vi "Send Message Log Ready String to Debug Client.vi"(8 "error in (no error)":errorcluster, 10 "DC_UID":T1, 11 "DS TCP Server in":refnum<class "DS TCP Server.lvclass">) -> (0 "error out":errorcluster, 3 "DS TCP Server out":refnum<class "DS TCP Server.lvclass">)   [LabVIEW 2017, in "DS TCP Server.lvlib" / "DS TCP Server.lvclass"]
uses:
  DS TCP Server.lvclass
  Common VIs/DC_UID.ctl
  C:/Program Files (x86)/National Instruments/LabVIEW 2017/vi.lib/addons/_Workers/Library/Classes/Worker/Worker.lvclass
  rqp_Send Data to Debug Client.ctl
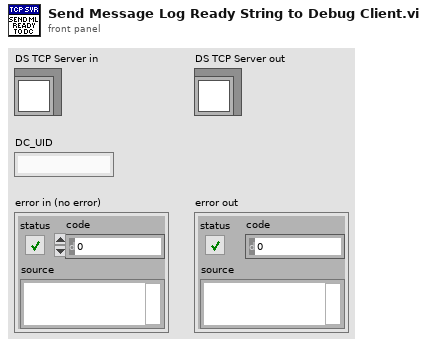
[diagram p1: front panel]
types:
  T1 = typedef "DC_UID.ctl" = string
  T2 = typedef "DS TCP Server.lvlib/DS TCP Server.lvclass/rqp_Send Data to Debug Client.ctl" = cluster{"DC_UID":T1, "String to send":string}
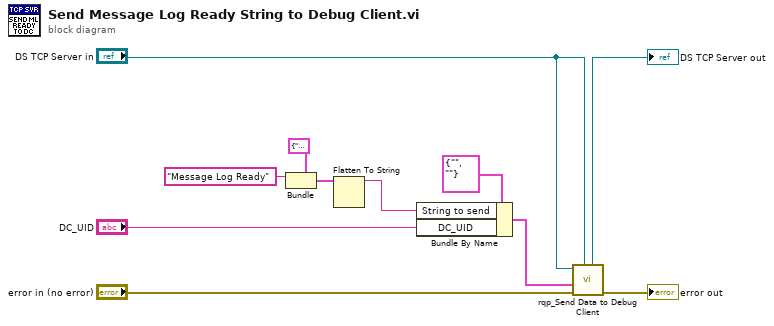
[diagram p0: block diagram]
diagram:
  n1 = Bundle(cluster=cluster{string, string} {"", ""}, "Message Log Ready") -> (w5:cluster{string, string})  [unwired: 1 in]
  n2 = Flatten To String(anything=w5) -> (data string=w9:string)  [unwired: 3 in, 2 out]
  n3 = Bundle By Name(cluster=T2 {"DC_UID"="", "String to send"=""} ("Data in"), "String to send"=w9, "DC_UID"="DC_UID") -> (w8:T2)
  n4 = call "rqp_Send Data to Debug Client.vi"("Caller in"="DS TCP Server in", "error in"="error in (no error)", "Data in"=w8, "DS TCP Server in"="DS TCP Server in") -> ("error out"=→"error out":errorcluster, "dup Caller out"=→"DS TCP Server out":refnum<class "DS TCP Server.lvclass">)  [unwired: 5 in, 1 out]
